vi "configure.vi"(8 "error in (no error)":errorcluster, 11 "WriteSignalsDAQmxPlugin in":refnum<class "SignalWriterMM140725DAQmx.lvclass">) -> (0 "error out":errorcluster, 3 "WriteSignalsDAQmxPlugin out":refnum<class "SignalWriterMM140725DAQmx.lvclass">)   [LabVIEW 2010, in "SignalWriterMM140725DAQmx.lvclass"]
uses:
  SignalWriterMM140725DAQmx.lvclass
  output_type_enum.ctl
  trigger_edge_enum.ctl
  common/classes/GenericComponent/GenericComponent/GenericComponent.lvclass
panel:
  in  "counter":tag
  out "configuration":string
  in  "edge":T1
  in  "digital trigger line":tag
  in  "output value upper bound":dbl caption="to"
  in  "output value  lower bound":dbl caption="from"
  in  "output type":T2
  in  "lag":dbl[unit]
  in  "timing source":tag
  in  "output physical channel":tag
  in  "cancel button":bool
  in  "save button":bool
  # "Configure DL090202DAQmxWriteSignals"
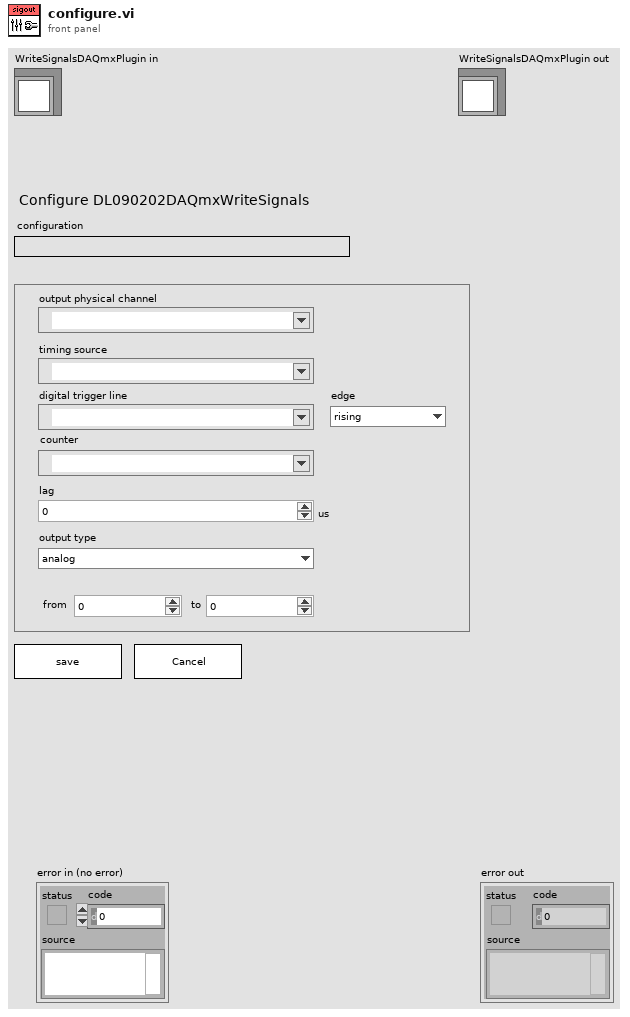
[diagram p1: front panel]
types:
  T1 = typedef "SignalWriterMM140725DAQmx.lvclass/trigger_edge_enum.ctl" = enum16{"rising", "falling"}
  T2 = typedef "SignalWriterMM140725DAQmx.lvclass/output_type_enum.ctl" = enum16{"analog", "digital (U8)", "digital (U16)", "digital (U32)"}
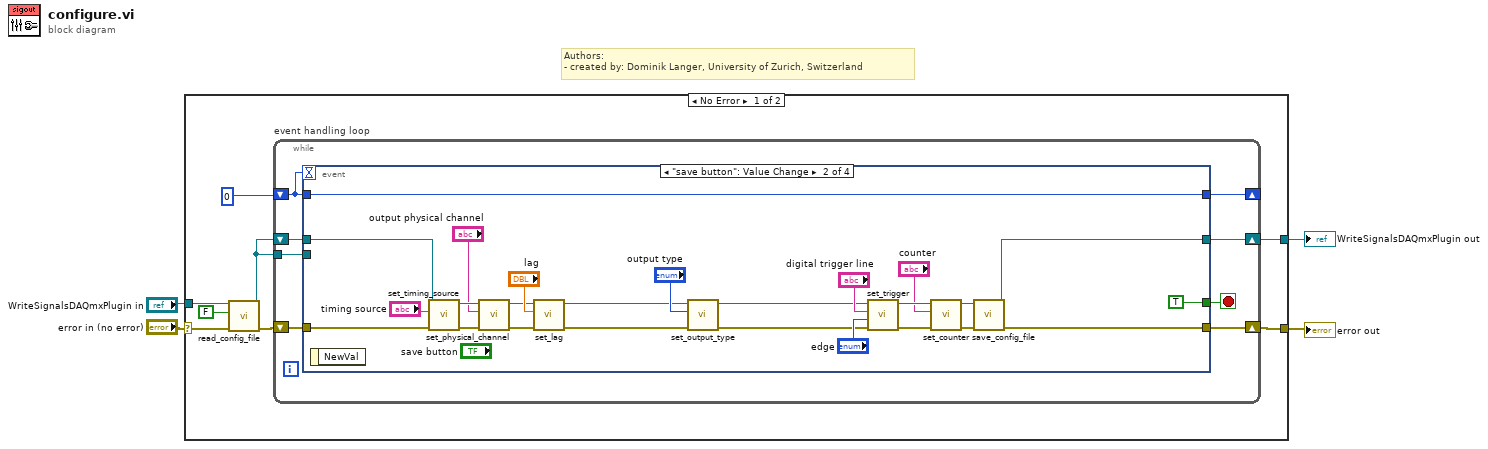
[diagram p0: block diagram]
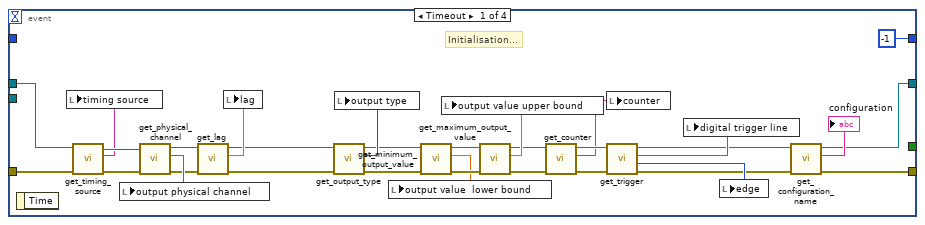
[diagram p2: hidden frame]
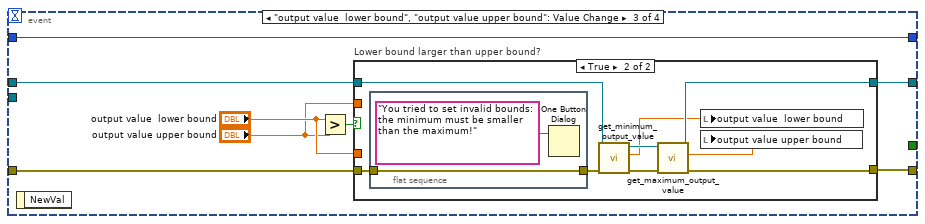
[diagram p3: hidden frame]
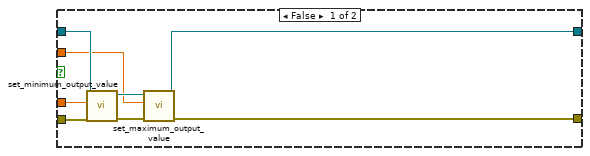
[diagram p4: hidden frame]
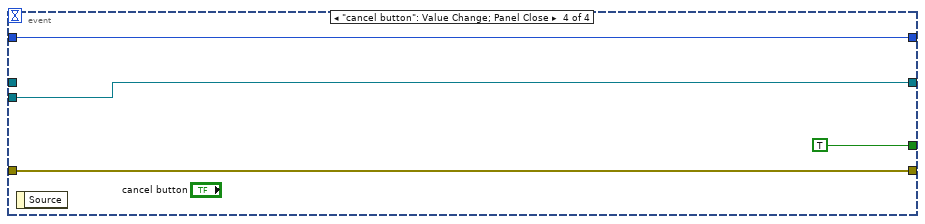
[diagram p5: hidden frame]
diagram:
  # "Authors: \n- created by: Dominik Langer, University of Zurich, Switzerland"
  n1 = case shown="No Error" "error in (no error)" {
    selector: "error in (no error)" -> [w8 w109]
    tunnel: [w12 w109] -> w3
    tunnel: [w10 w108] -> w1
    tunnel: "WriteSignalsDAQmxPlugin in" -> [w9 w108]
    frame No Error {
      n2 = call-dynamic "read_config_file.vi"("error in (no error)"=w8, "force load?"=FALSE, "GenericPlugin in"=w9) -> ("error out"=w7:errorcluster, "GenericPlugin out"=w5:refnum<class "SignalWriterMM140725DAQmx.lvclass">)  [unwired: 7 out]
      n3 = while "event handling loop" {
        shift-right: [w16] -> _
        shift-left: 0 -> [w17]
        shift-right: [w14] -> w10
        shift-left: w5 -> [w15]
        shift-right: [w19] -> w12
        shift-left: w7 -> [w20]
        tunnel: w5 -> [w13]
        stop <- w18 stop-if-true
        n4 = event shown="[1] \"save button\": Value Change" {
          selector: _ -> [_ _ _ _]
          dyn-events: _ -> [_ _ _ _]
          timeout: w17 -> [_ _ _ _]
          tunnel: w20 -> [w36 w73 w83 w106]
          tunnel: [w31 w64 w82 w106] -> w19
          tunnel: [_ TRUE _ TRUE] -> w18
          tunnel: [-1 w76 w84 w105] -> w16
          tunnel: w17 -> [_ w76 w84 w105]
          tunnel: w15 -> [w35 w72 w81 _]
          tunnel: [w28 w63 w80 w104] -> w14
          tunnel: w13 -> [_ _ _ w104]
          event Timeout {
            # "Initialisation..."
            n5 = event-data() -> ()  [unwired: 2 out]
            n6 = call-dynamic "get_timing_source.vi"("error in (no error)"=w36, "DAQmxWriteSignals.lvclass in"=w35) -> ("error out"=w49:errorcluster, "timing source"=w48:tag, "DAQmxWriteSignals.lvclass out"=w50:refnum<class "SignalWriterMM140725DAQmx.lvclass">)  [unwired: 7 out]
            n7 = local write "timing source"(w48) -> ()
            n8 = call-dynamic "get_physical_channel.vi"("error in (no error)"=w49, "DAQmxWriteSignals.lvclass in"=w50) -> ("error out"=w45:errorcluster, "physical channel"=w47:tag, "DAQmxWriteSignals.lvclass out"=w46:refnum<class "SignalWriterMM140725DAQmx.lvclass">)  [unwired: 7 out]
            n9 = local write "output physical channel"(w47) -> ()
            n10 = call-dynamic "get_lag.vi"("error in (no error)"=w45, "GenericWriteSignals.lvclass in"=w46) -> ("error out"=w22:errorcluster, "lag"=w44:dbl[unit], "GenericWriteSignals.lvclass out"=w21:refnum<class "SignalWriterMM140725DAQmx.lvclass">)  [unwired: 7 out]
            n11 = local write "lag"(w44) -> ()
            n12 = call-dynamic "get_output_type.vi"("error in (no error)"=w22, "DAQmxWriteSignals.lvclass in"=w21) -> ("error out"=w42:errorcluster, "output type"=w43:T2, "DAQmxWriteSignals.lvclass out"=w41:refnum<class "SignalWriterMM140725DAQmx.lvclass">)  [unwired: 7 out]
            n13 = local write "output type"(w43) -> ()
            n14 = call-dynamic "get_minimum_output_value.vi"("error in (no error)"=w42, "GenericWriteSignals.lvclass in"=w41) -> ("error out"=w40:errorcluster, "minimum output value"=w37:dbl, "GenericWriteSignals.lvclass out"=w39:refnum<class "SignalWriterMM140725DAQmx.lvclass">)  [unwired: 7 out]
            n15 = local write "output value  lower bound"(w37) -> ()
            n16 = call-dynamic "get_maximum_output_value.vi"("error in (no error)"=w40, "GenericWriteSignals.lvclass in"=w39) -> ("error out"=w27:errorcluster, "maximum output value"=w38:dbl, "GenericWriteSignals.lvclass out"=w25:refnum<class "SignalWriterMM140725DAQmx.lvclass">)  [unwired: 7 out]
            n17 = local write "output value upper bound"(w38) -> ()
            n18 = call-dynamic "get_counter.vi"("error in (no error)"=w27, "SignalWriterDL090202DAQmx in"=w25) -> ("error out"=w26:errorcluster, "counter"=w23:tag, "SignalWriterDL090202DAQmx out"=w24:refnum<class "SignalWriterMM140725DAQmx.lvclass">)  [unwired: 6 in, 1 out]
            n19 = local write "counter"(w23) -> ()
            n20 = call-dynamic "get_trigger.vi"("error in (no error)"=w26, "DAQmxWriteSignals in"=w24) -> ("error out"=w32:errorcluster, "edge"=w34:T1, "digital trigger line"=w33:tag, "DAQmxWriteSignals out"=w29:refnum<class "SignalWriterMM140725DAQmx.lvclass">)  [unwired: 6 out]
            n21 = local write "digital trigger line"(w33) -> ()
            n22 = local write "edge"(w34) -> ()
            n23 = call "get_configuration_name.vi"("error in (no error)"=w32, "GenericPlugin.lvclass in"=w29) -> ("error out"=w31:errorcluster, "configuration name"=→"configuration":string, "GenericPlugin.lvclass out"=w28:refnum<class "SignalWriterMM140725DAQmx.lvclass">)  [unwired: 7 in]
          }
          event "save button": Value Change {
            n24 = event-data() -> ()  [unwired: 2 out]
            n25 = call-dynamic "set_timing_source.vi"("error in (no error)"=w73, "timing source"="timing source", "DAQmxWriteSignals.lvclass in"=w72) -> ("error out"=w74:errorcluster, "DAQmxWriteSignals.lvclass out"=w71:refnum<class "SignalWriterMM140725DAQmx.lvclass">)  [unwired: 7 out]
            n26 = call-dynamic "set_physical_channel.vi"("error in (no error)"=w74, "physical channel"="output physical channel", "DAQmxWriteSignals.lvclass in"=w71) -> ("error out"=w68:errorcluster, "DAQmxWriteSignals.lvclass out"=w66:refnum<class "SignalWriterMM140725DAQmx.lvclass">)  [unwired: 7 out]
            n27 = call-dynamic "set_lag.vi"("error in (no error)"=w68, "lag"="lag", "DAQmxWriteSignals.lvclass in"=w66) -> ("error out"=w53:errorcluster, "DAQmxWriteSignals.lvclass out"=w52:refnum<class "SignalWriterMM140725DAQmx.lvclass">)  [unwired: 7 out]
            n28 = call-dynamic "set_output_type.vi"("error in (no error)"=w53, "output type"="output type", "DAQmxWriteSignals.lvclass in"=w52) -> ("error out"=w55:errorcluster, "DAQmxWriteSignals.lvclass out"=w54:refnum<class "SignalWriterMM140725DAQmx.lvclass">)  [unwired: 7 out]
            n29 = call-dynamic "set_trigger.vi"("error in (no error)"=w55, "edge"="edge", "digital trigger line"="digital trigger line", "DAQmxWriteSignals in"=w54) -> ("error out"=w60:errorcluster, "DAQmxWriteSignals out"=w58:refnum<class "SignalWriterMM140725DAQmx.lvclass">)  [unwired: 6 out]
            n30 = call-dynamic "set_counter.vi"("error in (no error)"=w60, "counter"="counter", "SignalWriterDL090202DAQmx in"=w58) -> ("error out"=w59:errorcluster, "SignalWriterDL090202DAQmx out"=w57:refnum<class "SignalWriterMM140725DAQmx.lvclass">)  [unwired: 7 in]
            n31 = call-dynamic "save_config_file.vi"("error in (no error)"=w59, "GenericPlugin in"=w57) -> ("error out"=w64:errorcluster, "GenericPlugin out"=w63:refnum<class "SignalWriterMM140725DAQmx.lvclass">)  [unwired: 2 in, 6 out]
          }
          event "output value  lower bound", "output value upper bound": Value Change {
            n32 = event-data() -> ()  [unwired: 2 out]
            n33 = Greater?(x="output value  lower bound", y="output value upper bound") -> (0:w79:bool)
            n34 = case "Lower bound larger than upper bound?" shown="True" w79 {
              tunnel: w83 -> [w91 w94]
              tunnel: [w89 w99] -> w82
              tunnel: w81 -> [w88 w98]
              tunnel: [w87 w97] -> w80
              tunnel: "output value  lower bound" -> [w86 _]
              tunnel: "output value upper bound" -> [w85 _]
              frame False {
                n35 = call-dynamic "set_minimum_output_value.vi"("error in (no error)"=w91, "minimum output value"=w86, "DAQmxWriteSignals.lvclass in"=w88) -> ("error out"=w90:errorcluster, "DAQmxWriteSignals.lvclass out"=w92:refnum<class "SignalWriterMM140725DAQmx.lvclass">)  [unwired: 7 out]
                n36 = call-dynamic "set_maximum_output_value.vi"("error in (no error)"=w90, "maximum output value"=w85, "DAQmxWriteSignals.lvclass in"=w92) -> ("error out"=w89:errorcluster, "DAQmxWriteSignals.lvclass out"=w87:refnum<class "SignalWriterMM140725DAQmx.lvclass">)  [unwired: 7 out]
              }
              frame True {
                n37 = flat-sequence {
                  tunnel: w94 -> [w103]
                  tunnel: [w103] -> w93
                  frame #0 {
                    n38 = One Button Dialog(message="You tried to set invalid bounds: the minimum must be smaller than the maximum!") -> ()  [unwired: 1 in, 1 out]
                  }
                }
                n39 = call-dynamic "get_minimum_output_value.vi"("error in (no error)"=w93, "GenericWriteSignals.lvclass in"=w98) -> ("error out"=w100:errorcluster, "minimum output value"=w96:dbl, "GenericWriteSignals.lvclass out"=w101:refnum<class "SignalWriterMM140725DAQmx.lvclass">)  [unwired: 7 out]
                n40 = call-dynamic "get_maximum_output_value.vi"("error in (no error)"=w100, "GenericWriteSignals.lvclass in"=w101) -> ("error out"=w99:errorcluster, "maximum output value"=w95:dbl, "GenericWriteSignals.lvclass out"=w97:refnum<class "SignalWriterMM140725DAQmx.lvclass">)  [unwired: 7 out]
                n41 = local write "output value  lower bound"(w96) -> ()
                n42 = local write "output value upper bound"(w95) -> ()
              }
            }
          }
          event "cancel button": Value Change; Panel Close {
            n43 = event-data() -> ()  [unwired: 2 out]
          }
        }
      }
    }
    frame Error {
    }
  }
  "error out" <- w3
  "WriteSignalsDAQmxPlugin out" <- w1
